vi "Test Post-filter.vi"(8 "error in (no error)":errorcluster, 11 "DSP.lvclass":refnum<class "DSP.lvclass">) -> (0 "error out":errorcluster, 3 "DSP.lvclass":refnum<class "DSP.lvclass">)   [LabVIEW 2019, in "DSP.lvclass"]
uses:
  DSP.lvclass
  Typedefs/REF.Channel--Cluster--Array.ctl
  Typedefs/REF.Channel--Cluster.ctl
  Typedefs/DSP.Config.Timing--Cluster.ctl
  DSP.lvclass/DSP.ctl
  <vilib>/Waveform/WDTOps.llb/WDT Append Waveforms DBL.vi
  Create Low Pass RC Filter (FGV).vi
  Create Low Pass Filter (FGV).vi
  DFD Filter Array.vi
  <vilib>/measure/maspectr.llb/FFT Power Spectrum and PSD for N Chan.vi
  <vilib>/measure/NI_MABase.lvlib
  <vilib>/measure/NI_MAPro.lvlib
panel:
  in  "Butterworth? [T]":bool=TRUE
  out "PS Waveform":cluster{"f0":dbl, "df":dbl, "magnitude":dbl[]}[](graph)
  out "phase out":dbl[](array[numeric])
  out "Waveform 2":waveform(dbl)[](graph)
  in  "frequency":dbl[](array[numeric]) format="%0.2p"
  in  "REF Channels 2":T1 {"Roll-Off" min=1; "TC" min=0.0001 format="%#_3p"; "Phase" format="%.3g"; "Frequency" min=0.0001 max=10000.0 format="%.3g"; "Channel" min=1}
  out "Waveform 1":waveform(dbl)[](graph)
  in  "stop":bool
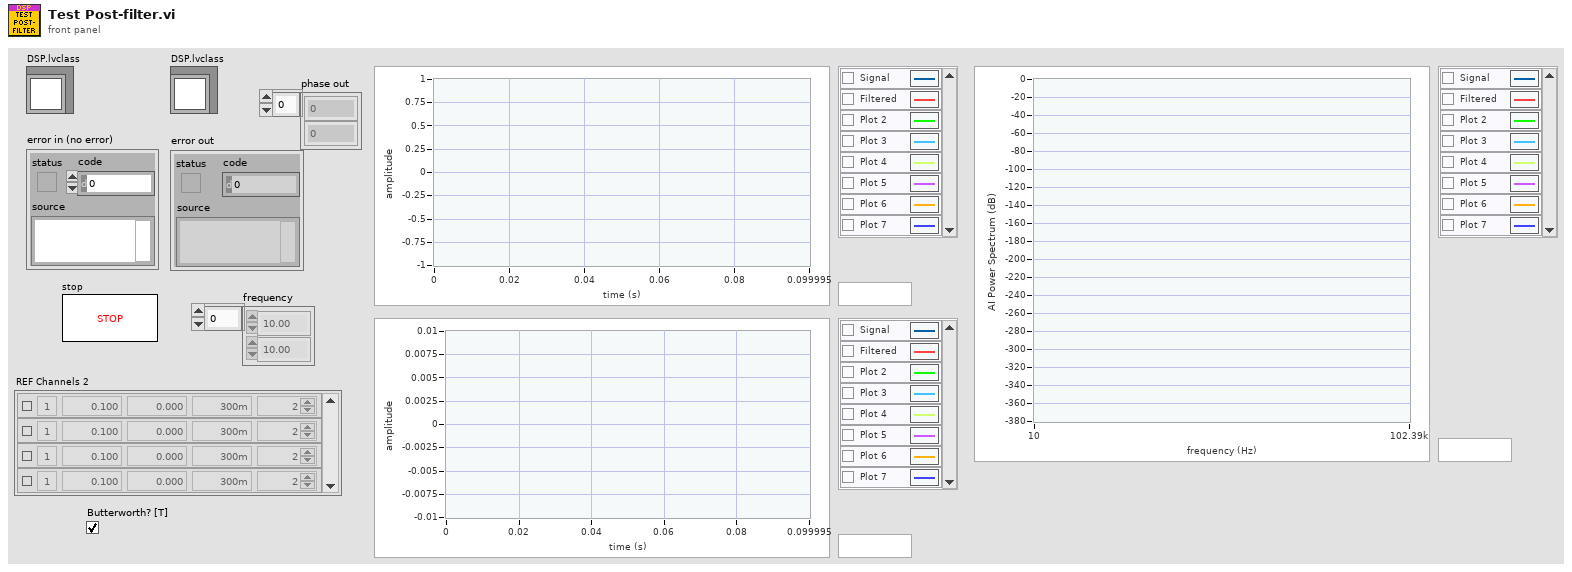
[diagram p1: front panel]
types:
  T1 = typedef "DSP.lvclass/REF.Channel--Cluster--Array.ctl" = T2[]
  T2 = typedef "DSP.lvclass/REF.Channel--Cluster.ctl" = cluster{"Enable?":bool, "Channel":i32, "Frequency":dbl, "Phase":dbl, "TC":dbl, "Roll-Off":i32}
  T3 = typedef "DSP.lvclass/DSP.Config.Timing--Cluster.ctl" = cluster{"Sampling":cluster{"Fs":dbl, "#s":i32}, "Fs_Out":dbl}
  T4 = enum16{"No averaging", "Vector averaging", "RMS averaging", "Peak hold"}
  T5 = cluster{"averaging mode":enum16{"No averaging", "Vector averaging", "RMS averaging", "Peak hold"}, "weighting mode":enum16{"Linear", "Exponential"}, "number of averages":u32}
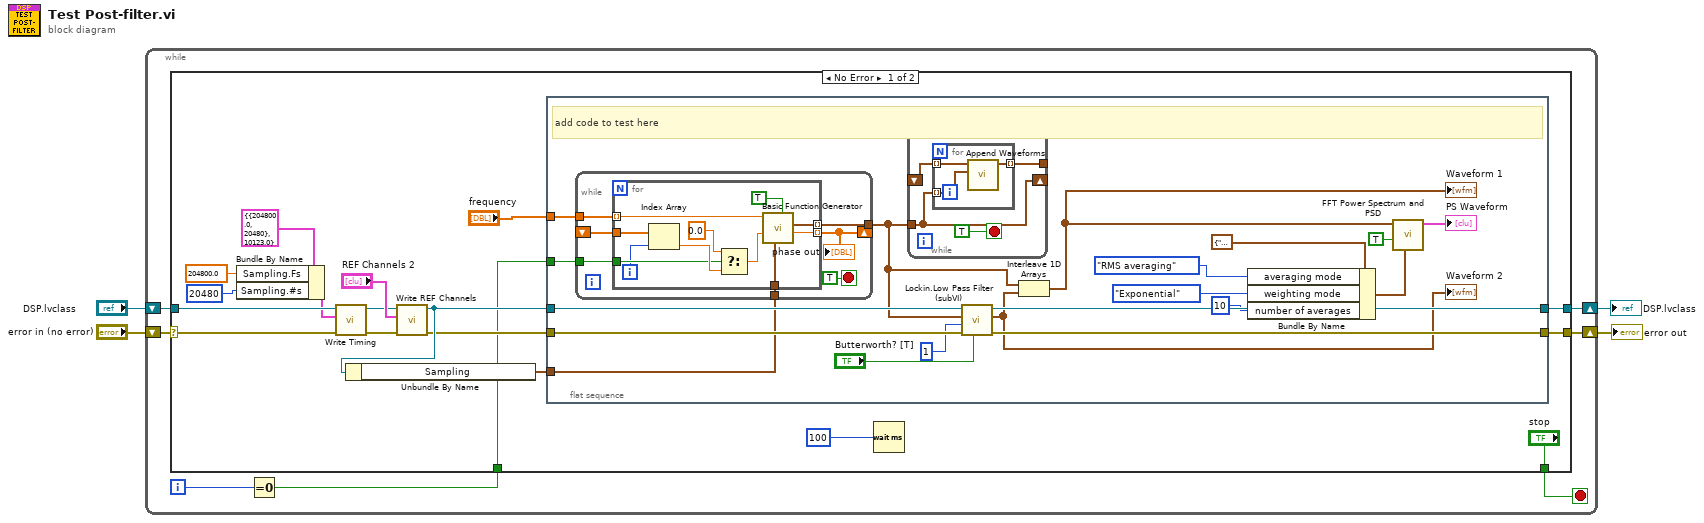
[diagram p0: block diagram]
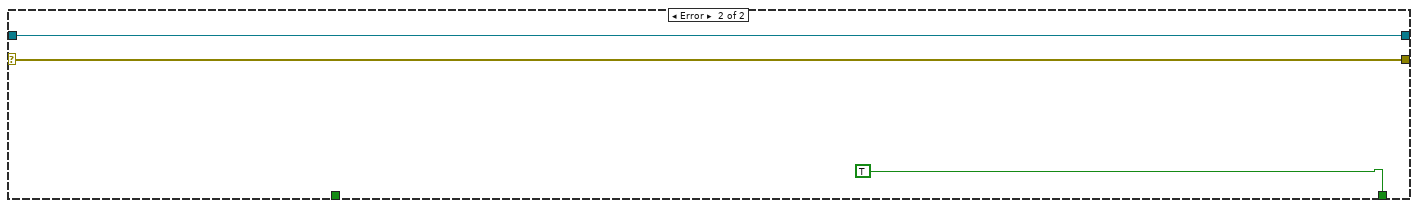
[diagram p2: hidden frame]
diagram:
  n1 = while {
    shift-right: [w10] -> w3
    shift-left: "error in (no error)" -> [w11]
    shift-right: [w8] -> w1
    shift-left: "DSP.lvclass" -> [w9]
    i -> [w7]
    stop <- w6 stop-if-true
    n2 = Equal To 0?(x=w7) -> (x = 0?=w5:bool)
    n3 = case shown="No Error" w11 {
      selector: w11 -> [w20 w76]
      tunnel: [w28 w76] -> w10
      tunnel: [w29 w75] -> w8
      tunnel: w9 -> [w21 w75]
      tunnel: ["stop" TRUE ("stop")] -> w6
      tunnel: w5 -> [w16 _]
      frame No Error {
        n4 = Bundle By Name(cluster=T3 {"Sampling"={"Fs"=204800.0, "#s"=20480}, "Fs_Out"=10123.0} ("Timing"), "Sampling.Fs"=204800.0, "Sampling.#s"=20480) -> (w12:T3)
        n5 = call "Write Timing.vi"("error in (no error)"=w20, "Timing"=w12, "DSP in"=w21) -> ("error out"=w19:errorcluster, "DSP out"=w22:refnum<class "DSP.lvclass">)  [unwired: 7 in]
        n6 = call "Write REF Channels.vi"("error in (no error)"=w19, "REF Channels"="REF Channels 2", "DSP in"=w22) -> ("error out"=w25:errorcluster, "DSP out"=w26:refnum<class "DSP.lvclass">)  [unwired: 7 in]
        n7 = Unbundle By Name(w26) -> ("Sampling"=w18:cluster{"Fs":dbl, "#s":i32})
        n8 = flat-sequence {
          tunnel: [w48] -> w29
          tunnel: w25 -> [w46]
          tunnel: [w47] -> w28
          tunnel: w26 -> [w43]
          tunnel: "frequency" -> [w44]
          tunnel: w18 -> [w42]
          tunnel: w16 -> [w41]
          frame #0 {
            # "add code to test here"
            n9 = while {
              tunnel: w44 -> [w62]
              tunnel: w42 -> [w61]
              tunnel: [w60] -> w40
              shift-right: [w59] -> _
              shift-left: _ -> [w58]
              tunnel: w41 -> [w56]
              stop <- TRUE stop-if-true
              n10 = for {
                tunnel: [w73] -> w60 mode=indexing
                tunnel: w62 -> [w72] mode=indexing
                tunnel: w61 -> [w71]
                tunnel: [w70] -> w59 mode=indexing
                tunnel: w58 -> [w69]
                tunnel: w56 -> [w64]
                i -> [w63]
                n11 = Index Array(array=w69, index=w63) -> (element=w66:dbl)
                n12 = Select(t=0.0, s=w64, f=w66) -> (s? t:f=w67:dbl)
                n13 = call <vilib>:"Basic Function Generator.vi"("reset signal"=TRUE, "sampling info"=w71, "phase"=w67, "frequency"=w72) -> ("phase out"=w70:dbl, "signal out"=w73:waveform(dbl))  [unwired: 5 in, 1 out]
              }
              "phase out" <- w59
            }
            n14 = while {
              tunnel: w40 -> [w50]
              shift-right: [w50] -> _
              shift-left: _ -> [w51]
              tunnel: [w49] -> _
              stop <- TRUE stop-if-true
              n15 = for {
                tunnel: w50 -> [w55] mode=indexing
                tunnel: [w54] -> w49 mode=indexing
                tunnel: w51 -> [w53] mode=indexing
                n16 = call-poly <vilib>:"Append Waveforms.vi"("waveform B"=w55, "waveform A"=w53) -> ("waveform out"=w54:waveform(dbl))  [unwired: 8 in, 1 out]
              }
            }
            n17 = call "Lockin.Low Pass Filter (subVI).vi"("Butterworth? [T]"="Butterworth? [T]", "error in (no error)"=w46, "Element Data"=1, "signal in"=w40, "DSP in"=w43) -> ("error out"=w47:errorcluster, "signal out"=w31:waveform(dbl)[], "DSP out"=w48:refnum<class "DSP.lvclass">)  [unwired: 3 in, 1 out]
            "Waveform 2" <- w31
            n18 = Interleave 1D Arrays(w40, w31) -> (w33:waveform(dbl)[])
            "Waveform 1" <- w33
            n19 = Bundle By Name(cluster=T5 {"averaging mode"=enum."No averaging", "weighting mode"=enum."Exponential", "number of averages"=10} ("averaging parameters"), "averaging mode"=T4."RMS averaging", "weighting mode"=enum16{"Linear", "Exponential"}."Exponential", "number of averages"=u32 10 ("# averages")) -> (w37:T5)
            n20 = call-poly <vilib>:"FFT Power Spectrum and PSD.vi"("averaging parameters"=w37, "dB On (F)"=TRUE, "time signals"=w33) -> ("Power Spectrum / PSD"=→"PS Waveform":cluster{"f0":dbl, "df":dbl, "magnitude":dbl[]}[])  [unwired: 5 in, 3 out]
          }
        }
        n21 = Wait (ms)(milliseconds to wait=u32 100) -> ()  [unwired: 1 out]
      }
      frame Error {
      }
    }
  }
  "error out" <- w3
  "DSP.lvclass" <- w1
